vi "cornell-K0edges.vi"(6 "Numeric":i32=500, 7 "secelt":T1, 8 "τ":dbl=1.0, 9 "h":dbl, 10 "s":dbl, 11 "ω":dbl) -> (0 "Ks(ω)":cdb)   [LabVIEW 2020]
uses:
  cornell-Ktildesh2sides.ctl
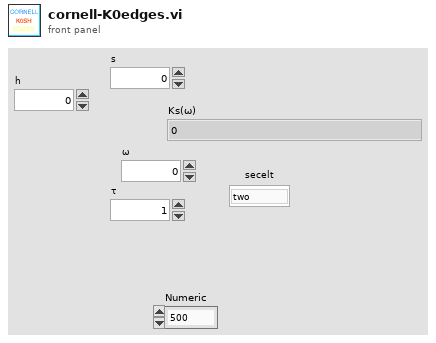
[diagram p1: front panel]
types:
  T1 = typedef "cornell-Ktildesh2sides.ctl" = enum16{"two", "one", "uni", "check1", "check2", "two½", "zcoth(z)", "z/sinh(z)", "one½", "brute"}
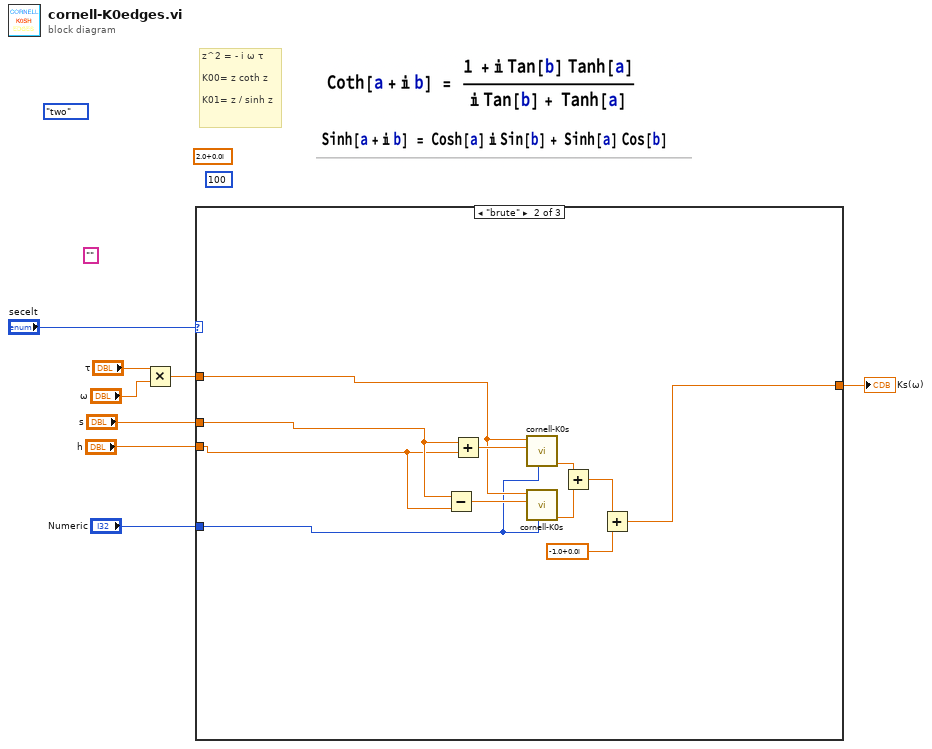
[diagram p0: block diagram]
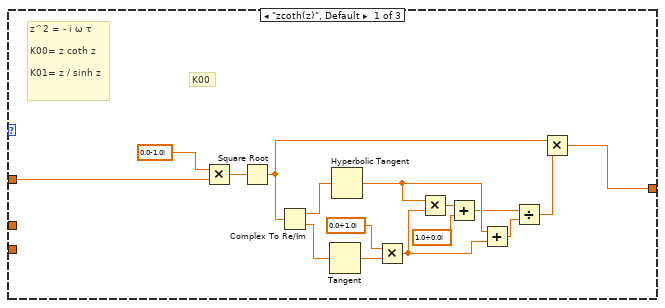
[diagram p2: hidden frame]
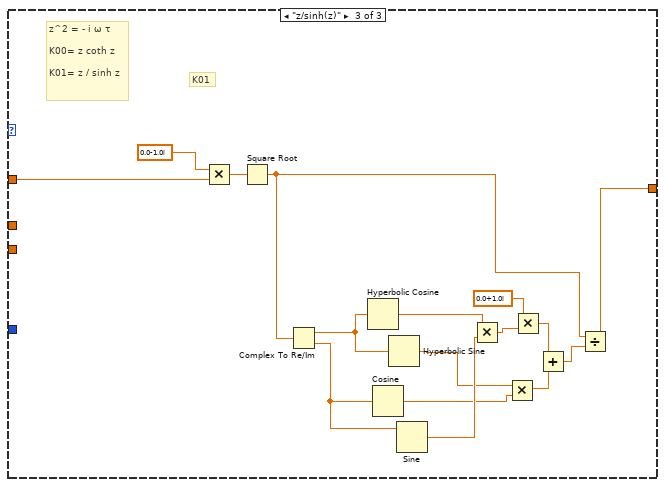
[diagram p3: hidden frame]
diagram:
  (unwired) cornell-Ktildesh2sides."two" ("Enum")
  (unwired) ""
  (unwired) cdb 2.0+0.0i
  (unwired) 100
  # "z^2 = - i ω τ\n\nK00= z coth z\n\nK01= z / sinh z"
  n1 = Multiply(x="τ", y="ω") -> (x*y=w4:dbl)
  n2 = case shown="\"brute\"" "secelt" {
    tunnel: "s" -> [_ w28 _]
    tunnel: "h" -> [_ w27 _]
    tunnel: w4 -> [w24 w29 w51]
    tunnel: [w9 w25 w36] -> w3
    tunnel: "Numeric" -> [_ w26 _]
    frame "zcoth(z)", Default {
      # "K00"
      # "z^2 = - i ω τ\n\nK00= z coth z\n\nK01= z / sinh z"
      n3 = Multiply(x=cdb 0.0-1.0i, y=w24) -> (x*y=w22:cdb)
      n4 = Square Root(x=w22) -> (sqrt(x)=w10:cdb)
      n5 = Complex To Re/Im(x + iy=w10) -> (x=w19:dbl, y=w18:dbl)
      n6 = Tangent(1:w18) -> (0:w21:dbl)
      n7 = Hyperbolic Tangent(1:w19) -> (0:w15:dbl)
      n8 = Multiply(x=cdb 0.0+1.0i, y=w21) -> (x*y=w14:cdb)
      n9 = Multiply(x=w15, y=w14) -> (x*y=w17:cdb)
      n10 = Add(x=w17, y=cdb 1.0+0.0i) -> (x+y=w12:cdb)
      n11 = Add(x=w15, y=w14) -> (x+y=w13:cdb)
      n12 = Divide(x=w12, y=w13) -> (x/y=w11:cdb)
      n13 = Multiply(x=w10, y=w11) -> (x*y=w9:cdb)
    }
    frame "brute" {
      n14 = Subtract(x=w28, y=w27) -> (x-y=w34:dbl)
      n15 = Add(x=w28, y=w27) -> (x+y=w35:dbl)
      n16 = call "cornell-K0s.vi"("Numeric"=w26, "s"=w35, "ω"=w29) -> ("Ks(ω)"=w33:cdb)  [unwired: 8 in]
      n17 = call "cornell-K0s.vi"("Numeric"=w26, "s"=w34, "ω"=w29) -> ("Ks(ω)"=w32:cdb)  [unwired: 8 in]
      n18 = Add(x=w33, y=w32) -> (x+y=w31:cdb)
      n19 = Add(x=w31, y=cdb -1.0+0.0i ("x")) -> (x+y=w25:cdb)
    }
    frame "z/sinh(z)" {
      # "K01"
      # "z^2 = - i ω τ\n\nK00= z coth z\n\nK01= z / sinh z"
      n20 = Multiply(x=cdb 0.0-1.0i, y=w51) -> (x*y=w49:cdb)
      n21 = Square Root(x=w49) -> (sqrt(x)=w38:cdb)
      n22 = Complex To Re/Im(x + iy=w38) -> (x=w48:dbl, y=w47:dbl)
      n23 = Hyperbolic Cosine(1:w48) -> (0:w46:dbl)
      n24 = Cosine(x=w47) -> (cos(x)=w41:dbl)
      n25 = Hyperbolic Sine(1:w48) -> (0:w42:dbl)
      n26 = Sine(x=w47) -> (sin(x)=w45:dbl)
      n27 = Multiply(x=w46, y=w45) -> (x*y=w43:dbl)
      n28 = Multiply(x=w42, y=w41) -> (x*y=w39:dbl)
      n29 = Multiply(x=cdb 0.0+1.0i, y=w43) -> (x*y=w40:cdb)
      n30 = Add(x=w40, y=w39) -> (x+y=w37:cdb)
      n31 = Divide(x=w38, y=w37) -> (x/y=w36:cdb)
    }
  }
  "Ks(ω)" <- w3
